vi "Add Add-Instrument to Tree.vi"(7 "ItemType":T1=enum."Add Thermometer", 8 "error in (no error)":errorcluster, 9 "#ofComparators (New ComparatorID)":i32, 10 "Instrument Group Tag in":string, 11 "TreeControl in":refnum<vi>) -> (0 "error out":errorcluster, 1 "Add Instrument Tag Out":string, 3 "TreeControl out":refnum<vi>)   [LabVIEW 2018]
uses:
  TypeDefs/Tree Item Type.ctl
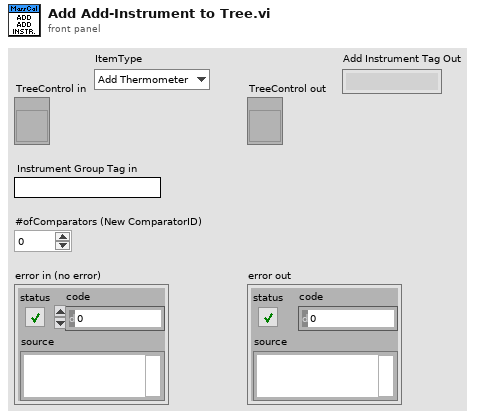
[diagram p1: front panel]
types:
  T1 = typedef "Tree Item Type.ctl" = enum16{"Comparator", "Temp Group", "Press Group", "Hygro Group", "Thermometer", "PressureTransducer", "Hygrometers", "Add Comparator", "Add Thermometer", "Add Barometer", "Add Hygrometer"}
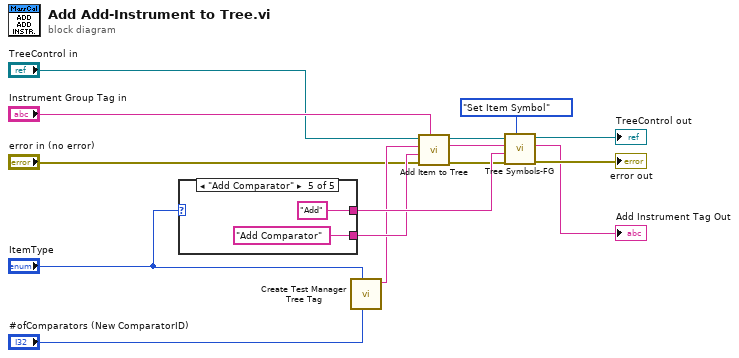
[diagram p0: block diagram]
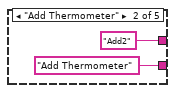
[diagram p3: hidden frame]
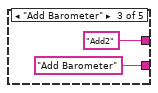
[diagram p4: hidden frame]
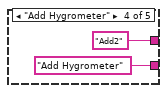
[diagram p5: hidden frame]
diagram:
  n1 = case shown="\"Add Comparator\"" "ItemType" {
    tunnel: [_ "Add2" ("Symbol Name") "Add2" ("Symbol Name") "Add2" ("Symbol Name") "Add" ("Symbol Name")] -> w12
    tunnel: [_ "Add Thermometer" ("Item Name") "Add Barometer" ("Item Name") "Add Hygrometer" ("Item Name") "Add Comparator" ("Item Name")] -> w6
    frame Default {
    }
    frame "Add Thermometer" {
    }
    frame "Add Barometer" {
    }
    frame "Add Hygrometer" {
    }
    frame "Add Comparator" {
    }
  }
  n2 = call "Create Test Manager Tree Tag.vi"("Comparator ID"="#ofComparators (New ComparatorID)", "ItemType"="ItemType") -> ("Tag"=w5:string)  [unwired: 7 in, 2 out]
  n3 = call "Add Item to Tree.vi"("Parent Tag"="Instrument Group Tag in", "error in (no error)"="error in (no error)", "Item Name"=w6, "Item Tag"=w5, "Tree Ref"="TreeControl in") -> ("error out"=w7:errorcluster, "Item Tag out"=w10:string, "reference out"=w8:refnum<vi>)  [unwired: 3 in, 1 out]
  n4 = call "Tree Symbols-FG.vi"("Actions"=enum16{"Init Symbols", "Set Item Symbol"}."Set Item Symbol", "error in (no error)"=w7, "Symbol Name"=w12, "Item Tag"=w10, "Tree Ref"=w8) -> ("error out"=→"error out":errorcluster, "Item Tag out"=→"Add Instrument Tag Out":string, "Tree Ref out"=→"TreeControl out":refnum<vi>)  [unwired: 4 in]
